vi "Enigma_rot.vi"(2 "Kiekon numero":i32, 3 "Kiekot sisään":string[][][](array[string])) -> (1 "Kiekot ulos":string[][][](array[string]))   [LabVIEW 2023]
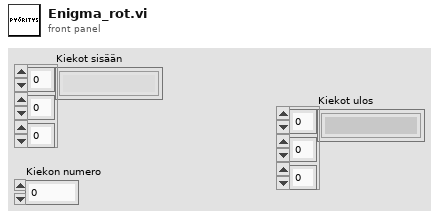
[diagram p1: front panel]
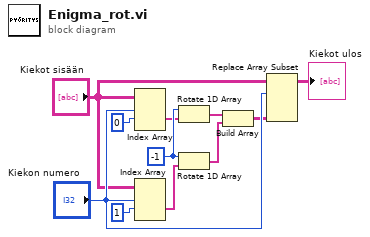
[diagram p0: block diagram]
diagram:
  w9 = -1 ("n")
  n1 = Index Array(array="Kiekot sisään", index (dim 0)="Kiekon numero", index (dim 1)=0 ("disabled index (row)")) -> (element=w5:string[])  [unwired: 1 in]
  n2 = Index Array(array="Kiekot sisään", index (dim 0)="Kiekon numero", index (dim 1)=1 ("disabled index (row)")) -> (element=w8:string[])  [unwired: 1 in]
  n3 = Rotate 1D Array(1:w5, 2:w9) -> (0:w11:string[])
  n4 = Rotate 1D Array(1:w8, 2:w9) -> (0:w10:string[])
  n5 = Build Array(w11, w10) -> (w2:string[][])
  n6 = Replace Array Subset(array="Kiekot sisään", new element=w2, index (dim 0)="Kiekon numero") -> (→"Kiekot ulos":string[][][])  [unwired: 2 in]
